vi "CC Get Channels.vi"(8 "error in (no error)":errorcluster, 11 "file path":path) -> (0 "error out":errorcluster, 3 "Channel List":T1[](array[typedef]))   [LabVIEW 2021]
uses:
  cluster CC Channel from TDMS.ctl
panel:
  out "group names":string[](array[string])
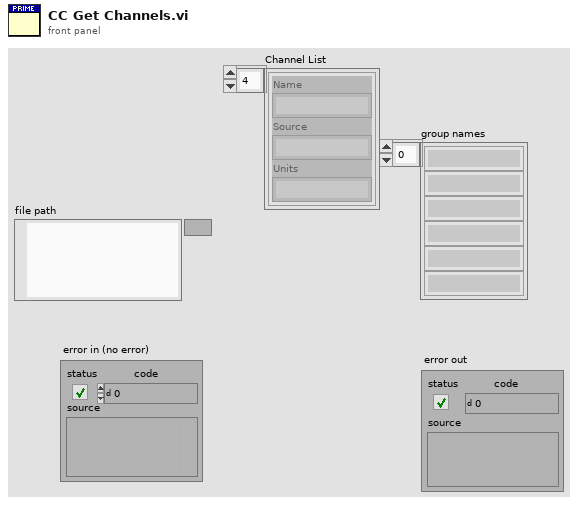
[diagram p1: front panel]
types:
  T1 = typedef "cluster CC Channel from TDMS.ctl" = cluster{"Name":string, "Source":string, "Units":string}
  T2 = enum16{"open", "open or create", "create or replace", "create", "open (read-only)"}
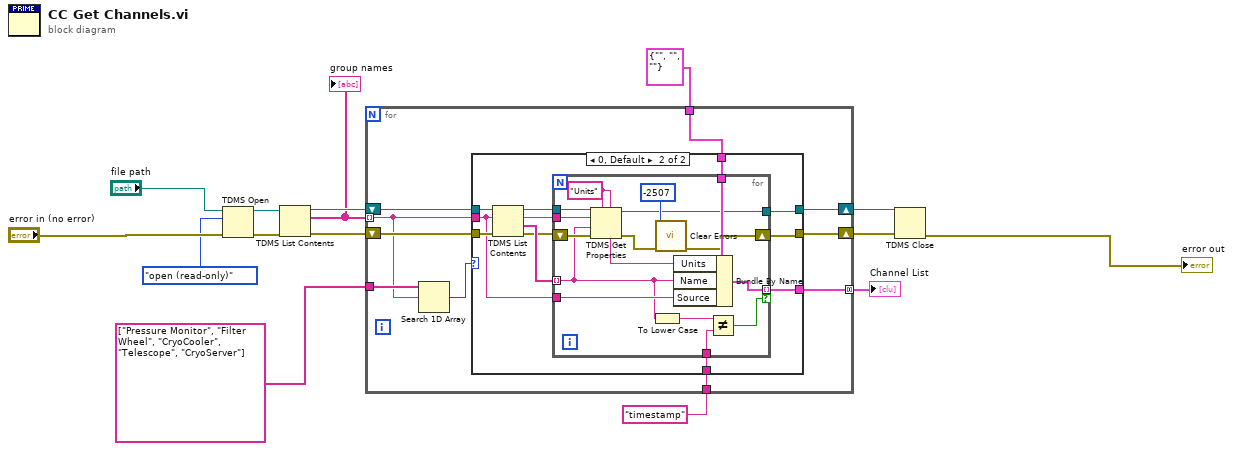
[diagram p0: block diagram]
diagram:
  n1 = TDMS Open(8:"error in (no error)", 10:T2."open (read-only)" ("operation (0:open)"), 11:"file path") -> (0:w12:errorcluster, 3:w11:refnum<k34>)  [unwired: 4 in]
  n2 = TDMS List Contents(4:w12, 7:w11) -> (0:w9:errorcluster, 2:w5:string[], 3:w8:refnum<k34>)  [unwired: 1 in, 1 out]
  "group names" <- w5
  n3 = for {
    shift-right: [w24] -> w6
    shift-left: w9 -> [w25]
    shift-right: [w22] -> w7
    shift-left: w8 -> [w23]
    tunnel: w5 -> [w17] mode=indexing
    tunnel: T1 {"Name"="", "Source"="", "Units"=""} -> [w21]
    tunnel: [w20] -> w3 mode=concatenating
    tunnel: "timestamp" ("regular expression") -> [w19]
    tunnel: string[] ["Pressure Monitor", "Filter Wheel", "CryoCooler", "Telescope", "CryoServer"] ("group names") -> [w18]
    n4 = Search 1D Array(1D array=w18, element=w17) -> (index of element=w16:i32)  [unwired: 1 in]
    n5 = case shown="0, Default" w16 {
      tunnel: w25 -> [w26 w39]
      tunnel: [w26 w28] -> w24
      tunnel: w23 -> [w27 w38]
      tunnel: [w27 w30] -> w22
      tunnel: w21 -> [_ w37]
      tunnel: w17 -> [_ w36]
      tunnel: [_ w34] -> w20
      tunnel: w19 -> [_ w33]
      frame -1 {
      }
      frame 0, Default {
        n6 = TDMS List Contents(4:w39, 6:w36, 7:w38) -> (0:w32:errorcluster, 1:w35:string[], 2:w29:string, 3:w31:refnum<k34>)
        n7 = for {
          tunnel: w37 -> [w55]
          tunnel: w36 -> [w54]
          tunnel: w35 -> [w47] mode=indexing
          tunnel: [w53] -> w34 mode=indexing if=w50
          tunnel: w33 -> [w51]
          shift-right: [w41] -> w28
          shift-left: w32 -> [w49]
          tunnel: w31 -> [w48]
          tunnel: [w42] -> w30
          tunnel: w29 -> [w40]
          w46 = "Units" ("property name")
          n8 = TDMS Get Properties(5:w46, 7:w46, 8:w49, 9:w47, 10:w40, 11:w48) -> (0:w43:errorcluster, 3:w42:refnum<k34>, 4:w45:string)  [unwired: 3 out]
          n9 = To Lower Case(string=w47) -> (all lower case string=w52:string)
          n10 = call <vilib>:"Clear Errors.vi"("error in (no error)"=w43, "specific error code to clear (0: all)"=-2507) -> ("error out"=w41:errorcluster)  [unwired: 4 in, 1 out]
          n11 = Bundle By Name(cluster=w55, "Units"=w45, "Name"=w47, "Source"=w54) -> (w53:T1)
          n12 = Not Equal?(x=w52, y=w51) -> (x != y?=w50:bool)
        }
      }
    }
  }
  "Channel List" <- w3
  n13 = TDMS Close(8:w6, 11:w7) -> (0:→"error out":errorcluster)  [unwired: 1 out]
